vi "Test_SQLQueryVIMSTR_WorksNoError.vi"(8 "error in (no error)":errorcluster, 11 "TestCase in":refnum<class "Test mysql.lvclass">) -> (0 "error out":errorcluster, 3 "TestCase out":refnum<class "Test mysql.lvclass">)   [LabVIEW 2020, in "DataBase_mysql_Tests.lvlib" / "Test mysql.lvclass"]
uses:
  Test mysql.lvclass
  98ffd0c8-4361-48ce-8721-6d705661544a.vi
  <vilib>/Utility/error.llb/Error Cluster From Error Code.vi
  externals/mysql/Source/mysql.net/mysql.lvclass
  <vilib>/addons/_JKI Toolkits/VI Tester/TestCase.llb/TestCase.lvclass
  C:/Program Files/National Instruments/LabVIEW 2020/vi.lib/addons/_JKI Toolkits/VI Tester/TestCase.llb/TestCase.lvclass
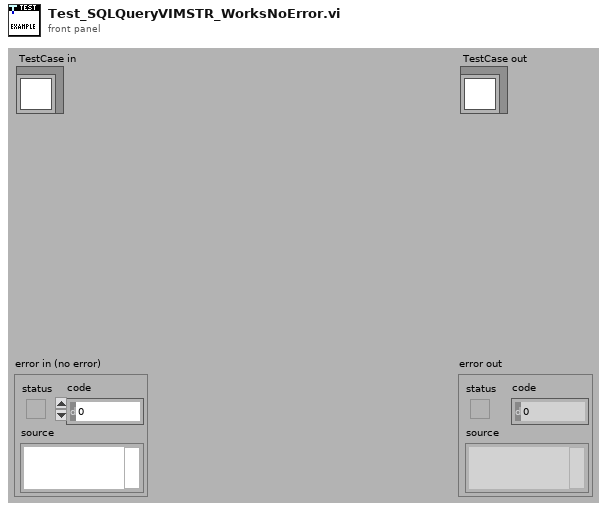
[diagram p1: front panel]
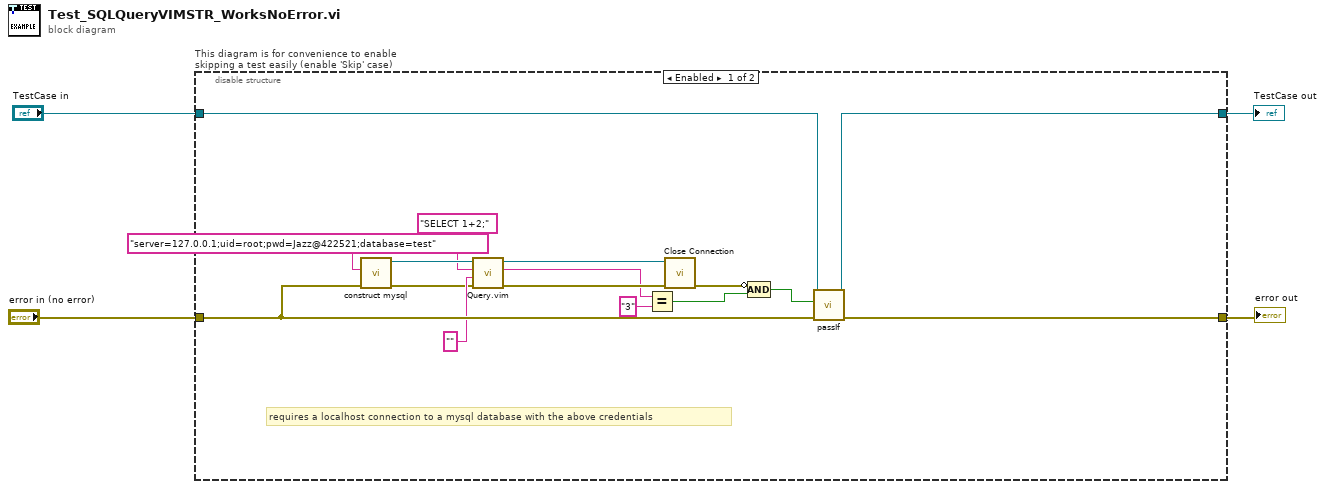
[diagram p0: block diagram]
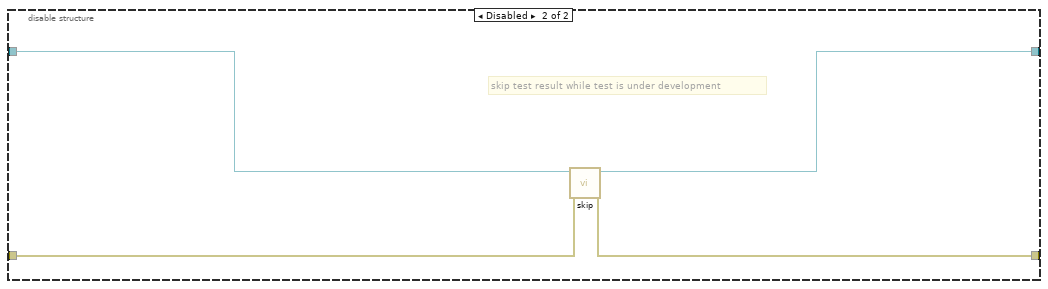
[diagram p2: hidden frame]
diagram:
  n1 = disable-structure "This diagram is for convenience to enable skipping a test easily (enable 'Skip' case)" shown="Enabled" {
    disable-tunnel: "TestCase in" -> [w20 w24]
    disable-tunnel: [w19 w22] -> w1
    disable-tunnel: [w18 w23] -> w3
    disable-tunnel: "error in (no error)" -> [w16 w21]
    frame Enabled {
      # "requires a localhost connection to a mysql database with the above credentials"
      n2 = call "construct mysql.vi"("error in (no error)"=w16, "Connection string"="server=127.0.0.1;uid=root;pwd=Jazz@422521;database=test") -> ("error out"=w5:errorcluster, "mysql out"=w11:refnum<class "mysql.lvclass">)  [unwired: 8 in]
      n3 = call "Query.vim"("error in (no error)"=w5, "Type and Default"="", "Query string"="SELECT 1+2;", "IDatabase in"=w11) -> ("error out"=w9:errorcluster, "Result"=w6:string, "IDatabase out"=w10:refnum<class "mysql.lvclass">)  [unwired: 5 in]
      n4 = Equal?(x=w6, y="3") -> (x = y?=w12:bool)
      n5 = call-dynamic "Close Connection.vi"("error in (no error)"=w9, "mysql in"=w10) -> ("error out"=w15:errorcluster)  [unwired: 8 in, 1 out]
      n6 = Compound Arithmetic op=AND(invert w15, w12) -> (w14:bool)
      n7 = call-dynamic "passIf.vi"("error in (no error)"=w16, "pass"=w14, "TestCase in"=w20) -> ("error out"=w18:errorcluster, "TestCase out"=w19:refnum<class "Test mysql.lvclass">)  [unwired: 7 in]
    }
    frame Disabled {
      # "skip test result while test is under development"
      n8 = call <vilib>:"skip.vi"("error in (no error)"=w21, "TestCase in"=w24) -> ("error out"=w23:errorcluster, "TestCase out"=w22:refnum<class "Test mysql.lvclass">)  [unwired: 8 in]
    }
  }
  "error out" <- w3
  "TestCase out" <- w1
